vi "STM Set Meta Data (UDP Ref).vi"(7 "Meta data":T1[](array[typedef]), 8 "error in":errorcluster, 11 "connection ID":refnum<k16>) -> (0 "error out":errorcluster, 3 "Connection Info Out":T2)   [LabVIEW 2010]
doc: "Assigns the meta data cluster associated with this STM session."
uses:
  stm_UDP Connection Info.ctl
  stm_MetaDataElement.ctl
  NI STM.lvlib
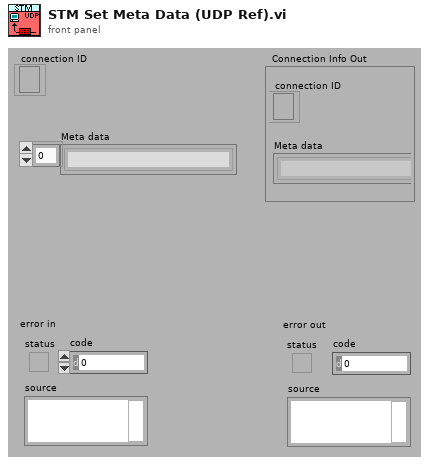
[diagram p1: front panel]
types:
  T1 = typedef "stm_MetaDataElement.ctl" = string
  T2 = typedef "stm_UDP Connection Info.ctl" = cluster{"connection ID":refnum<k16>, "Meta data":T1[]}
  T3 = typedef "NI STM.lvlib/UDP Connection Info.ctl" = cluster{"connection ID":refnum<k16>, "Meta data":T4[]}
  T4 = typedef "NI STM.lvlib/MetaDataElement.ctl" = string
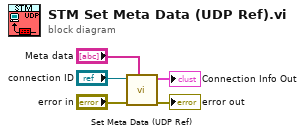
[diagram p0: block diagram]
diagram:
  n1 = call "Set Meta Data (UDP Ref).vi"("Meta data"="Meta data", "error in"="error in", "connection ID"="connection ID") -> ("error out"=→"error out":errorcluster, "Connection Info Out"=→"Connection Info Out":T3)  [unwired: 7 in]
